vi "Init.vi"(8 "error in (no error)":errorcluster, 11 "reference in":refnum<class "SwitchBase.lvclass">) -> (0 "error out":errorcluster, 3 "reference out":refnum<class "SwitchBase.lvclass">)   [LabVIEW 2022 SP3, in "SwitchBase.lvlib" / "SwitchBase.lvclass"]
uses:
  SwitchBase.lvclass
  Components/ViPER.lvlibp/ViPER.lvclass
  C:/Projects/Medulla/ViPER/Examples/Flux_Capacitor_Tester/Components/ViPER.lvlibp/ViPER.lvclass
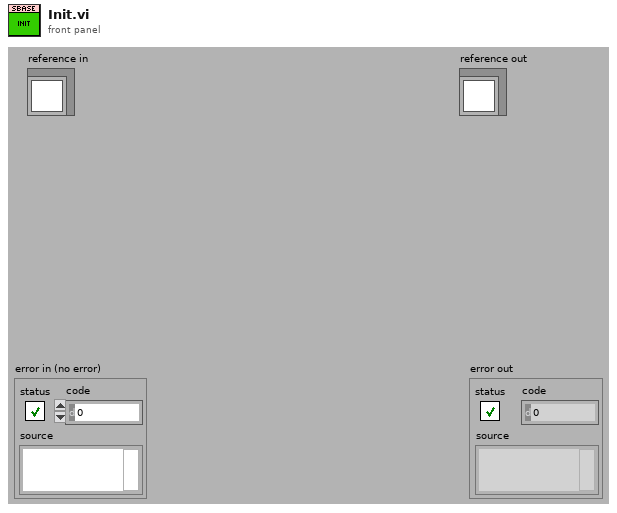
[diagram p1: front panel]
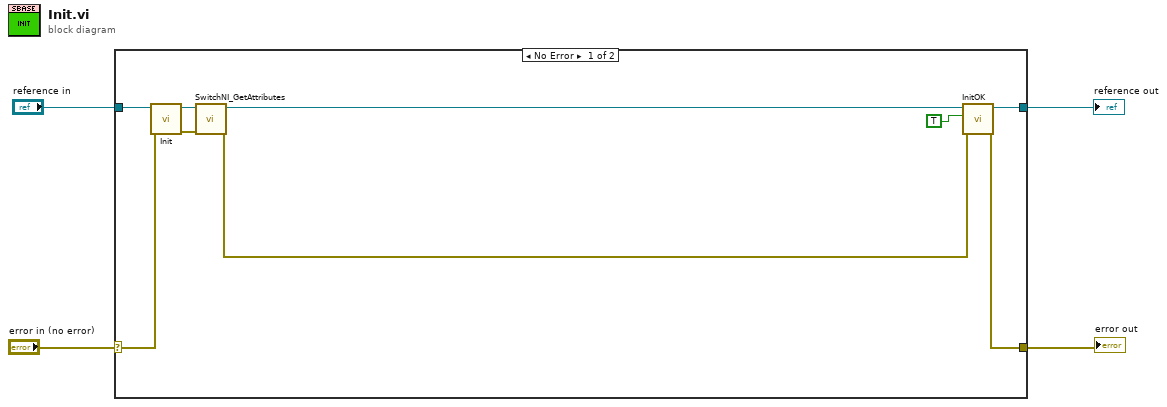
[diagram p0: block diagram]
diagram:
  n1 = case shown="No Error" "error in (no error)" {
    selector: "error in (no error)" -> [w12 w15]
    tunnel: [w6 w15] -> w3
    tunnel: [w8 w14] -> w1
    tunnel: "reference in" -> [w13 w14]
    frame No Error {
      n2 = call-parent "Init.vi"("error in (no error)"=w12, "reference in"=w13) -> ("error out"=w10:errorcluster, "reference out"=w11:refnum<class "SwitchBase.lvclass">)  [unwired: 8 in]
      n3 = call "SwitchNI_GetAttributes.vi"("error in (no error)"=w10, "reference in"=w11) -> ("error out"=w5:errorcluster, "reference out"=w9:refnum<class "SwitchBase.lvclass">)  [unwired: 6 in, 2 out]
      n4 = call "InitOK.vi"("error in (no error)"=w5, "Init OK?"=TRUE, "reference in"=w9) -> ("error out"=w6:errorcluster, "reference out"=w8:refnum<class "SwitchBase.lvclass">)  [unwired: 7 in]
    }
    frame Error {
    }
  }
  "error out" <- w3
  "reference out" <- w1
